vi "medicaoIXV.vi"() -> ()   [LabVIEW 2012]
uses:
  <vilib>/Utility/file.llb/Write To Spreadsheet File (string).vi
  <vilib>/Utility/file.llb/Write To Spreadsheet File (DBL).vi
  <instrlib>/Agilent 6XXX Series/Agilent 6XXX Series.lvlib
panel:
  in  "Tab Control":enum32{"Entrada de dados", "Saída de dados"}(tab)
  out "ON/OFF":bool
  in  "Pontos":dbl
  in  "Tensão máxima":dbl
  in  "Nome da célula":string
  in  "Local":path
  in  "Delay(s)":dbl
  in  "Start":bool
  out "IXV":cluster{"Y":dbl[], "Y":dbl[]}[](graph)
  out "output voltage":dbl
  out "Tensao Atual":dbl
  out "Corrente Atual":dbl
  out "Ponto Atual":i32
  out "TABELA DE DADOS\nTensão(fonte)     Tensão                  Corrente            Pontos":dbl[][](array[numeric]) caption="all rows" format="%0.3f"
  in  "CorrenteGraph":dbl
  in  "error in (no error)":errorcluster
  out "error out":errorcluster
  in  "TensaoGraph":dbl
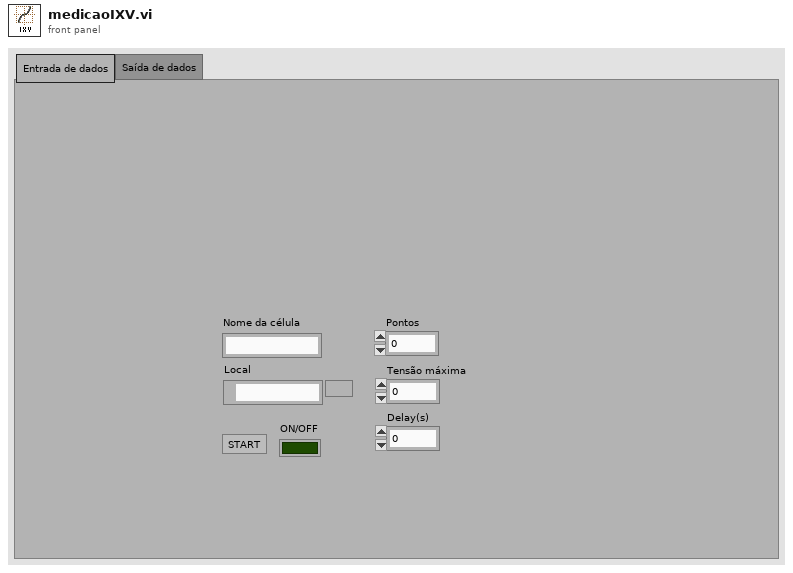
[diagram p1: front panel]
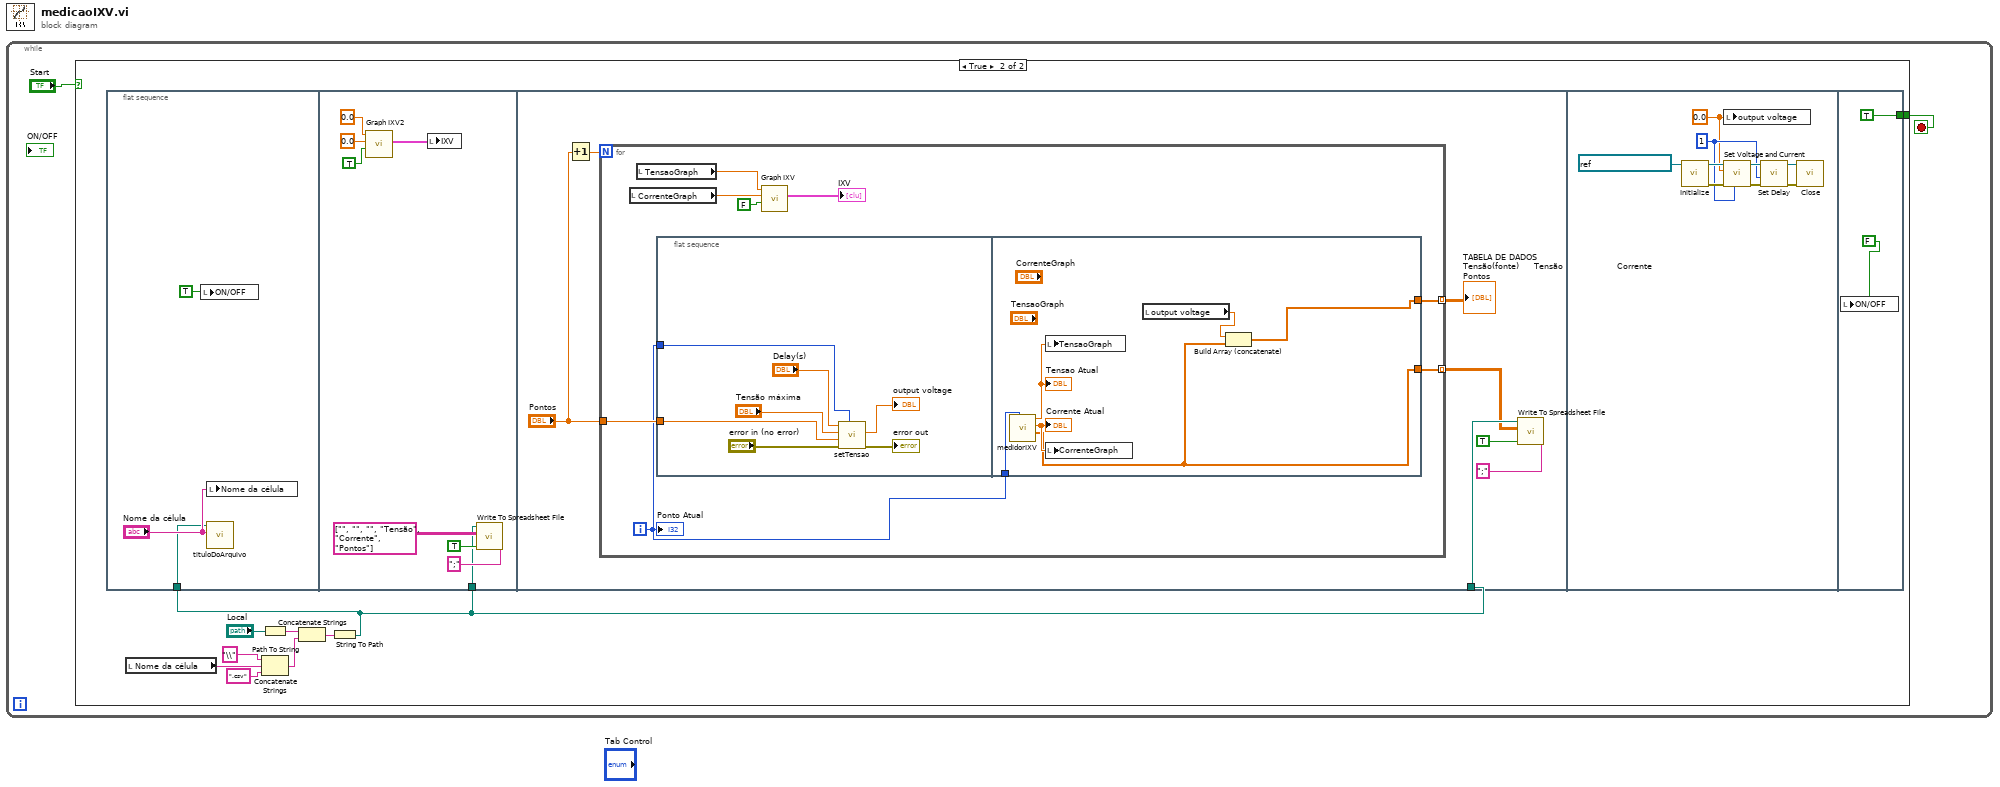
[diagram p0: block diagram]
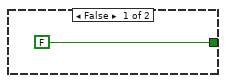
[diagram p2: hidden frame]
diagram:
  n1 = while {
    stop <- w1 stop-if-true
    n2 = case shown="True" "Start" {
      tunnel: [FALSE w6] -> w1
      frame False {
      }
      frame True {
        n3 = flat-sequence {
          tunnel: w4 -> [w14]
          tunnel: w4 -> [w20]
          tunnel: w4 -> [w28]
          tunnel: [TRUE] -> w6
          frame #0 {
            n4 = local write "ON/OFF"(TRUE ("ON/OFF")) -> ()
            n5 = local write "Nome da célula"("Nome da célula") -> ()
            n6 = call "tituloDoArquivo.vi"("Nome da célula"="Nome da célula", "file path (dialog if empty)"=w14) -> ()  [unwired: 10 in]
          }
          frame #1 {
            n7 = call "Graph IXV2"("Reset"=TRUE, "Y Input"=0.0, "X Input"=0.0) -> ("XY Graph"=w16:cluster{"Y":dbl[], "Y":dbl[]}[])  [unwired: 2 in, 6 out]
            n8 = local write "IXV"(w16) -> ()
            n9 = call-poly <vilib>:"Write To Spreadsheet File.vi"("delimiter (\\t)"=";" ("delimiter (\\t)"), "append to file? (new file:F)"=TRUE, "2D data"=string[][] [["", "", ""], ["Tensão", "Corrente", "Pontos"]], "file path (dialog if empty)"=w20) -> ()  [unwired: 4 in, 1 out]
          }
          frame #2 {
            n10 = Increment(x="Pontos") -> (x+1=w27:dbl)
            n11 = for {
              N: w27 -> [_]
              tunnel: [w32] -> w25 mode=indexing
              tunnel: "Pontos" -> [w38]
              tunnel: [w31] -> w24 mode=indexing
              i -> [w37]
              n12 = local read "CorrenteGraph"() -> (w36:dbl)
              n13 = local read "TensaoGraph"() -> (w35:dbl)
              n14 = flat-sequence {
                tunnel: w38 -> [w41]
                tunnel: w37 -> [w42]
                tunnel: [w48] -> w32
                tunnel: w37 -> [w51]
                tunnel: [w46] -> w31
                frame #0 {
                  n15 = call "setTensao.vi"("Ponto"=w42, "error in (no error)"="error in (no error)", "Pontos"=w41, "Tensão máxima"="Tensão máxima", "delay(s)"="Delay(s)") -> ("error out"=→"error out":errorcluster, "output voltage"=→"output voltage":dbl)  [unwired: 5 in]
                }
                frame #1 {
                  n16 = call "medidorIXV.vi"("Ponto"=w51) -> ("Array"=w48:dbl[], "Corrente Atual"=w50:dbl, "Tensao Atual"=w49:dbl)  [unwired: 8 in]
                  "Corrente Atual" <- w50
                  "Tensao Atual" <- w49
                  n17 = local write "TensaoGraph"(w49) -> ()
                  n18 = local write "CorrenteGraph"(w50) -> ()
                  n19 = local read "output voltage"() -> (w47:dbl)
                  n20 = Build Array (concatenate)(w47, w48) -> (w46:dbl[])
                }
              }
              n21 = call "Graph IXV"("Reset"=FALSE, "Y Input"=w36, "X Input"=w35) -> ("XY Graph"=→"IXV":cluster{"Y":dbl[], "Y":dbl[]}[])  [unwired: 2 in, 6 out]
              "Ponto Atual" <- w37
            }
            "TABELA DE DADOS\nTensão(fonte)     Tensão                  Corrente            Pontos" <- w24
            n22 = call-poly <vilib>:"Write To Spreadsheet File.vi"("delimiter (\\t)"=";" ("delimiter (\\t)"), "append to file? (new file:F)"=TRUE, "2D data"=w25, "file path (dialog if empty)"=w28) -> ()  [unwired: 4 in, 1 out]
          }
          frame #3 {
            w52 = 0.0 ("voltage (0 V)")
            w55 = u8 1 ("channel (1)")
            n23 = call <instrlib>:"Initialize.vi"("VISA resource name"=refnum<visa-resource-name> "GPIB0::5::INSTR") -> ("error out"=w57:errorcluster, "VISA resource name out"=w56:refnum<visa-resource-name>)  [unwired: 9 in]
            n24 = local write "output voltage"(w52) -> ()
            n25 = call <instrlib>:"Set Voltage and Current.vi"("channel (1)"=w55, "error in (no error)"=w57, "voltage (0 V)"=w52, "VISA resource name"=w56) -> ("error out"=w58:errorcluster, "VISA resource name out"=w59:refnum<visa-resource-name>)  [unwired: 6 in]
            n26 = call <instrlib>:"Set Delay.vi"("error in (no error)"=w58, "channel (1)"=w55, "VISA resource name"=w59) -> ("error out"=w53:errorcluster, "VISA resource name out"=w54:refnum<visa-resource-name>)  [unwired: 7 in]
            n27 = call <instrlib>:"Close.vi"("error in (no error)"=w53, "VISA resource name"=w54) -> ()  [unwired: 9 in, 1 out]
          }
          frame #4 {
            n28 = local write "ON/OFF"(FALSE) -> ()
          }
        }
        n29 = local read "Nome da célula"() -> (w7:string)
        n30 = Path To String(path="Local") -> (string=w11:string)
        n31 = Concatenate Strings("\\", w7, ".csv") -> (w12:string)
        n32 = Concatenate Strings(w11, w12) -> (w10:string)
        n33 = String To Path(string=w10) -> (path=w4:path)
      }
    }
  }
